vi "Check if the all actuators are in Home Position.vi"(8 "error in":errorcluster, 11 "UTP IO Session in":T1) -> (0 "error out":errorcluster, 2 "System is Ready?":bool, 3 "UTP IO Session out":T1)   [LabVIEW 2023, in "Actuators.lvlib"]
doc: "Check if the system is in Home Position"
uses:
  Actuators.lvlib
  <vilib>/Noffz/UTP IO/UTP IO Library/Typedefs/Session Handle.ctl
  <vilib>/Noffz/UTP IO/UTP IO Library/UTP IO Pool Session.lvclass
  <vilib>/Noffz/UTP IO/UTP IO Library/methods/poly/plc/Read PLC Variable (Boolean).vi
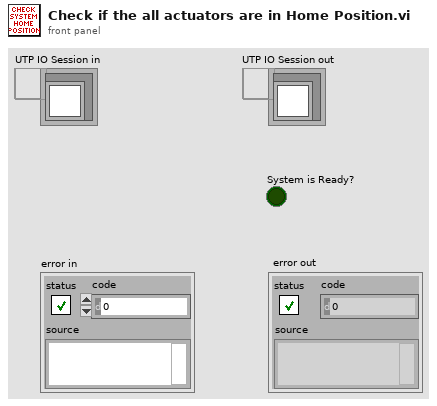
[diagram p1: front panel]
types:
  T1 = typedef "UTP IO Library.lvlib/UTP IO Pool Session.lvclass/Session Handle.ctl" = refnum<data-value>
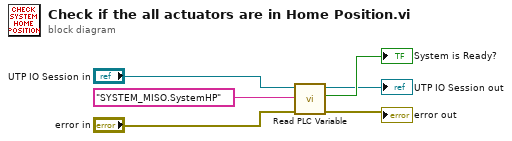
[diagram p0: block diagram]
diagram:
  n1 = call-poly <vilib>:"Read PLC Variable.vi"("error in (no error)"="error in", "variable name"="SYSTEM_MISO.SystemHP", "UTP IO Session in"="UTP IO Session in") -> ("error out"=→"error out":errorcluster, "value"=→"System is Ready?":bool, "UTP IO Session out"=→"UTP IO Session out":T1)  [unwired: 6 in]
